vi "Scalar JSON text to Variant (from Void).vi"(8 "error in (no error)":errorcluster, 10 "Offset":i32, 11 "JSON":string) -> (0 "error out":errorcluster, 1 "Variant out":variant)   [LabVIEW 2017, in "JSONtext.lvlib"]
uses:
  JSONtext.lvlib
  <vilib>/Utility/Data Type/Type Definitions/Data Type.ctl
  Advance past String.vi
  String Subset.vi
  support/Strip Quotes and Unescape.vi
  support/Get LVObject.vi
  support/Get Timestamp.vi
  support/Get I32.vi
  support/Get I64.vi
  support/Get U32.vi
  support/Get U64.vi
  support/Get Boolean.vi
  support/Get DBL.vi
  support/Get SGL.vi
  Advance past whitespace.vi
  support/Format Error.vi
  support/Get Number Text.vi
  NaN or null to Integer ERROR.vi
  Advance past Number.vi
  Parsing Error.vi
  <vilib>/Utility/error.llb/Error Cluster From Error Code.vi
  <vilib>/Utility/Data Type/Get Type Information.vi
  <vilib>/Utility/Data Type/Get Numeric Information.vi
  support/Unescape JSON string.vi
  support/Scan Timestamp.vi
  <vilib>/Utility/Data Type/Get Refnum Information.vi
  <vilib>/Utility/GetType.llb/TD_Create Cluster.vi
  <vilib>/LabVIEW Open Source Project/Data Manipulation/TypeDescriptor/TypeDescriptor_SetName.vi
  <vilib>/Utility/Data Type/NI_Data Type.lvlib
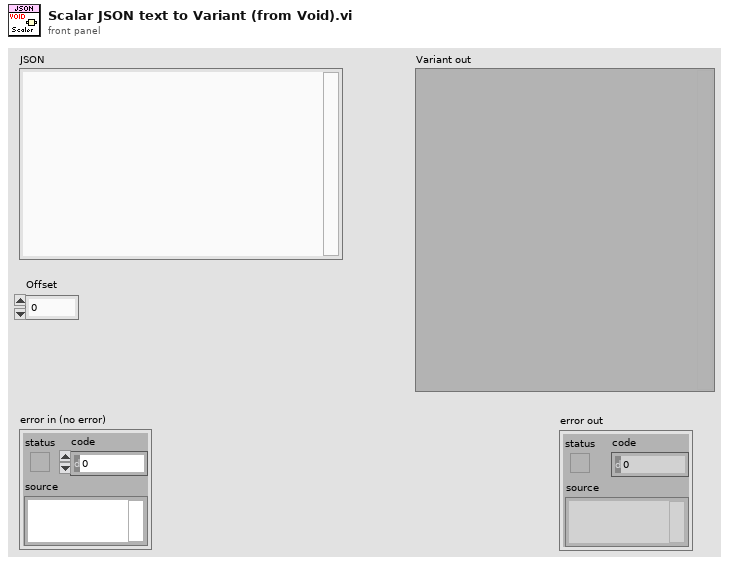
[diagram p1: front panel]
types:
  T1 = typedef "JSONtext.lvlib/JSON Value Type.ctl" = enum16{"Not a JSON Value", "JSON Object", "JSON Array", "String", "Number", "true", "false", "null"}
  T2 = typedef "NI_Data Type.lvlib/Data Type.ctl" = enum8{"Invalid Type", "Void", "I8", "I16", "I32", "I64", "U8", "U16", "U32", "U64", "Single Float", "Double Float", "Extended Float", "Single Complex", "Double Complex", "Extended Complex", "Enum U8", "Enum U16", "Enum U32", "Enum U64", "Single Float With Unit", "Double Float With Unit", "Extended Float With Unit", "Single Complex with Unit", "Double Complex with Unit", "Extended Complex with Unit", "Boolean", "String", "Path", "Picture", "Tag", "Array", "Cluster", "Variant", "LV Variant", "Waveform", "Timestamp", "Digital Waveform", "Digital Data", "ExpressData", "Refnum", "External Data", "VI", "Poly VI", "LabVIEW Class Instance", "Fixed Point"}
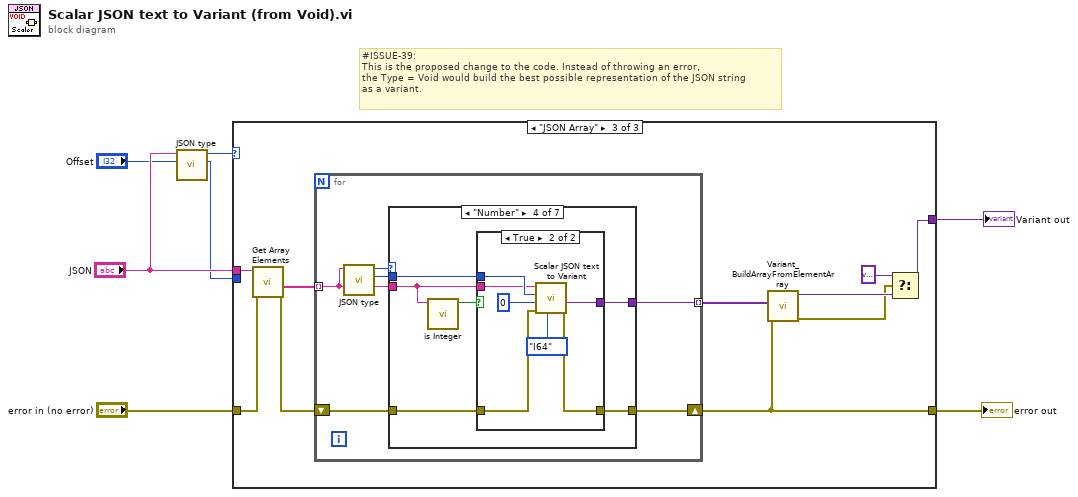
[diagram p0: block diagram]
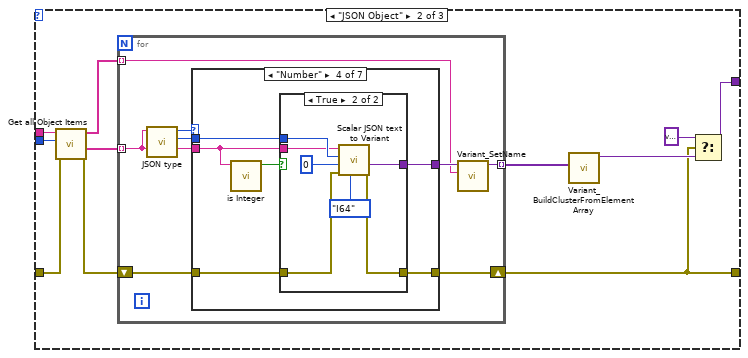
[diagram p3: hidden frame]
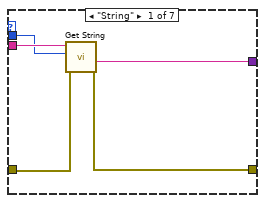
[diagram p4: hidden frame]
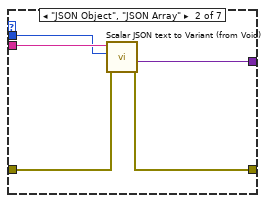
[diagram p5: hidden frame]
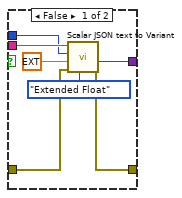
[diagram p7: hidden frame]
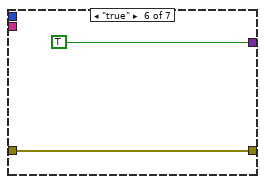
[diagram p9: hidden frame]
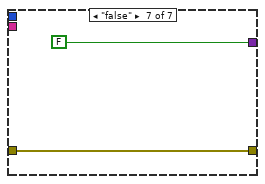
[diagram p10: hidden frame]
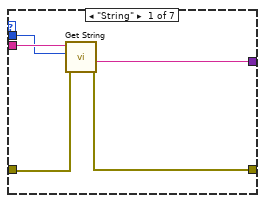
[diagram p11: hidden frame]
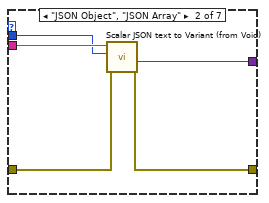
[diagram p12: hidden frame]
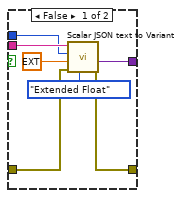
[diagram p14: hidden frame]
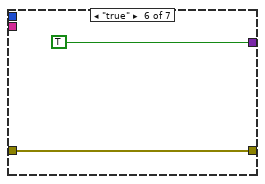
[diagram p16: hidden frame]
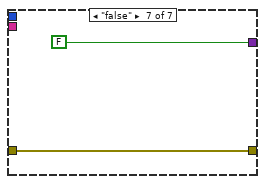
[diagram p17: hidden frame]
diagram:
  # "#ISSUE-39:\nThis is the proposed change to the code. Instead of throwing an error,\nthe Type = Void would build the best possible representation of the JSON string\nas a variant."
  n1 = call "JSON type.vi"("Offset"="Offset", "JSON"="JSON") -> ("Item Offset"=w3:i32, "JSON Value Type"=w2:T1)  [unwired: 8 in]
  n2 = case shown="\"JSON Array\"" w2 {
    tunnel: "error in (no error)" -> [w8 w11 w65]
    tunnel: [w8 w9 w69] -> w7
    tunnel: [_ w12 w70] -> w6
    tunnel: "JSON" -> [_ w19 w68]
    tunnel: w3 -> [_ w18 _]
    frame Default {
    }
    frame "JSON Object" {
      n3 = call "Get all Object Items.vi"("error in (no error)"=w11, "Offset"=w18, "JSON"=w19) -> ("error out"=w10:errorcluster, "<JSON>"=w16:string[], "Item Names"=w17:string[])  [unwired: 5 in, 1 out]
      n4 = for {
        tunnel: [w20] -> w15 mode=indexing
        tunnel: w17 -> [w21] mode=indexing
        tunnel: w16 -> [w23] mode=indexing
        shift-right: [w26] -> w9
        shift-left: w10 -> [w27]
        n5 = call "JSON type.vi"("JSON"=w23) -> ("Item Offset"=w24:i32, "JSON Value Type"=w25:T1)  [unwired: 9 in]
        n6 = case shown="\"Number\"" w25 {
          tunnel: [w28 w34 _ w41 _ TRUE FALSE] -> w22
          tunnel: w27 -> [w29 w33 w38 w43 w59 w60 w62]
          tunnel: [w30 w37 w38 w44 w59 w60 w62] -> w26
          tunnel: w23 -> [w32 w36 _ w40 _ _ _]
          tunnel: w24 -> [w31 w35 _ w42 _ _ _]
          frame "String" {
            n7 = call "Get String.vi"("error in (no error)"=w29, "Offset"=w31, "JSON"=w32) -> ("error out"=w30:errorcluster, "String"=w28:string)  [unwired: 6 in, 1 out]
          }
          frame "JSON Object", "JSON Array" {
            n8 = call "Scalar JSON text to Variant (from Void).vi"("error in (no error)"=w33, "Offset"=w35, "JSON"=w36) -> ("error out"=w37:errorcluster, "Variant out"=w34:variant)  [unwired: 7 in]
          }
          frame "null" {
          }
          frame "Number" {
            n9 = call "is Integer.vi"("<JSON>"=w40) -> ("is Integer?"=w39:bool)  [unwired: 10 in]
            n10 = case shown="True" w39 {
              tunnel: [w49 w57] -> w44
              tunnel: w43 -> [w48 w55]
              tunnel: w42 -> [w46 w53]
              tunnel: w40 -> [w51 w52]
              tunnel: [w50 w58] -> w41
              frame False {
                n11 = call "Scalar JSON text to Variant.vi"("Type"=Data_Type."Extended Float", "error in (no error)"=w48, "Variant (Data Type)"=ext 0.0, "Offset"=w46, "JSON"=w51) -> ("error out"=w49:errorcluster, "Variant out"=w50:variant)  [unwired: 5 in]
              }
              frame True {
                n12 = call "Scalar JSON text to Variant.vi"("Type"=Data_Type."I64", "error in (no error)"=w55, "Variant (Data Type)"=i64 0, "Offset"=w53, "JSON"=w52) -> ("error out"=w57:errorcluster, "Variant out"=w58:variant)  [unwired: 5 in]
              }
            }
          }
          frame "Not a JSON Value" {
          }
          frame "true" {
          }
          frame "false" {
          }
        }
        n13 = call "Variant_SetName.vi"("Name"=w21, "Variant"=w22) -> ("Named Variant"=w20:variant)  [unwired: 9 in]
      }
      n14 = call "Variant_BuildClusterFromElementArray.vi"("Elements"=w15) -> ("Cluster"=w13:variant)  [unwired: 10 in]
      n15 = Select(t=variant ("type"), s=w9, f=w13) -> (s? t:f=w12:variant)
    }
    frame "JSON Array" {
      n16 = call "Get Array Elements.vi"("error in (no error)"=w65, "JSON"=w68) -> ("error out"=w64:errorcluster, "<JSON>"=w67:string[])  [unwired: 7 in, 1 out]
      n17 = for {
        tunnel: [w74] -> w73 mode=indexing
        tunnel: w67 -> [w75] mode=indexing
        shift-right: [w78] -> w69
        shift-left: w64 -> [w79]
        n18 = call "JSON type.vi"("JSON"=w75) -> ("Item Offset"=w76:i32, "JSON Value Type"=w77:T1)  [unwired: 9 in]
        n19 = case shown="\"Number\"" w77 {
          tunnel: [w80 w86 _ w93 _ TRUE FALSE] -> w74
          tunnel: w79 -> [w81 w85 w90 w95 w111 w112 w114]
          tunnel: [w82 w89 w90 w96 w111 w112 w114] -> w78
          tunnel: w75 -> [w84 w88 _ w92 _ _ _]
          tunnel: w76 -> [w83 w87 _ w94 _ _ _]
          frame "String" {
            n20 = call "Get String.vi"("error in (no error)"=w81, "Offset"=w83, "JSON"=w84) -> ("error out"=w82:errorcluster, "String"=w80:string)  [unwired: 6 in, 1 out]
          }
          frame "JSON Object", "JSON Array" {
            n21 = call "Scalar JSON text to Variant (from Void).vi"("error in (no error)"=w85, "Offset"=w87, "JSON"=w88) -> ("error out"=w89:errorcluster, "Variant out"=w86:variant)  [unwired: 7 in]
          }
          frame "null" {
          }
          frame "Number" {
            n22 = call "is Integer.vi"("<JSON>"=w92) -> ("is Integer?"=w91:bool)  [unwired: 10 in]
            n23 = case shown="True" w91 {
              tunnel: [w101 w109] -> w96
              tunnel: w95 -> [w100 w107]
              tunnel: w94 -> [w98 w105]
              tunnel: w92 -> [w103 w104]
              tunnel: [w102 w110] -> w93
              frame False {
                n24 = call "Scalar JSON text to Variant.vi"("Type"=Data_Type."Extended Float", "error in (no error)"=w100, "Variant (Data Type)"=ext 0.0, "Offset"=w98, "JSON"=w103) -> ("error out"=w101:errorcluster, "Variant out"=w102:variant)  [unwired: 5 in]
              }
              frame True {
                n25 = call "Scalar JSON text to Variant.vi"("Type"=Data_Type."I64", "error in (no error)"=w107, "Variant (Data Type)"=i64 0, "Offset"=w105, "JSON"=w104) -> ("error out"=w109:errorcluster, "Variant out"=w110:variant)  [unwired: 5 in]
              }
            }
          }
          frame "Not a JSON Value" {
          }
          frame "true" {
          }
          frame "false" {
          }
        }
      }
      n26 = call "Variant_BuildArrayFromElementArray.vi"("error in (no error)"=w69, "Elements"=w73) -> ("error out"=w66:errorcluster, "Output Array"=w71:variant)  [unwired: 8 in]
      n27 = Select(t=variant ("type"), s=w66, f=w71) -> (s? t:f=w70:variant)
    }
  }
  "Variant out" <- w6
  "error out" <- w7
